vi "B Spline Fitting Demo.vi"() -> ()   [LabVIEW 2023]
doc: "This example generates data sets and then uses the B-Spline Fit VI (or its subVI) to create a best fit curve for the data. A best fit curve is generated each time you change the value of any of the controls."
uses:
  <vilib>/Native 3D Graph/xcontrol/3DPC_SurfacePlot.xctl
  <vilib>/Analysis/1siggen.llb/Ramp Pattern by Samples.vi
  <vilib>/Analysis/6fits.llb/1D B-Spline Fit.vi
  <vilib>/Analysis/6fits.llb/nD B-Spline Fit.vi
  <vilib>/Analysis/NI_AALBase.lvlib
  <vilib>/Analysis/NI_AALPro.lvlib
panel:
  in  "example selector":T1(tab)
  in  "parameter selection":u16(ring)=2 items=["equally spaced", "chord length", "centripetal"]
  in  "degree":i32=3
  in  "# of control points":i32=10
  out "1D B-Spline Fit on Arbitrary Curve":T2(graph)
  in  "# of control points":i32=30
  in  "degree":i32=7
  in  "parameter selection":u16(ring)=2 items=["equally spaced", "chord length", "centripetal"]
  in  "noise amplitude":dbl=0.01
  out "1D B-Spline Fit on Square Curve":T2(graph)
  out "B-Spline Fitted Curve":refnum<class "Base Datatype.lvclass">[](xcontrol)
  out "Original Curve":refnum<class "Base Datatype.lvclass">[](xcontrol)
  in  "noise amplitude":dbl=0.5
  in  "parameter selection":u16(ring)=2 items=["equally spaced", "chord length", "centripetal"]
  in  "degree":i32=3
  in  "# of control points":i32=15
  # "Overview: Demonstrates fitting curves with the B-Spline Fit VI.\nRequirements: LabVIEW Full Development System\nInstructions:\n1. Select a tab to specify which kind of fit to perform on which curve.\n2. Run the VI and observe the fit displayed on the graph.\n3. Select a different tab and run the VI again."
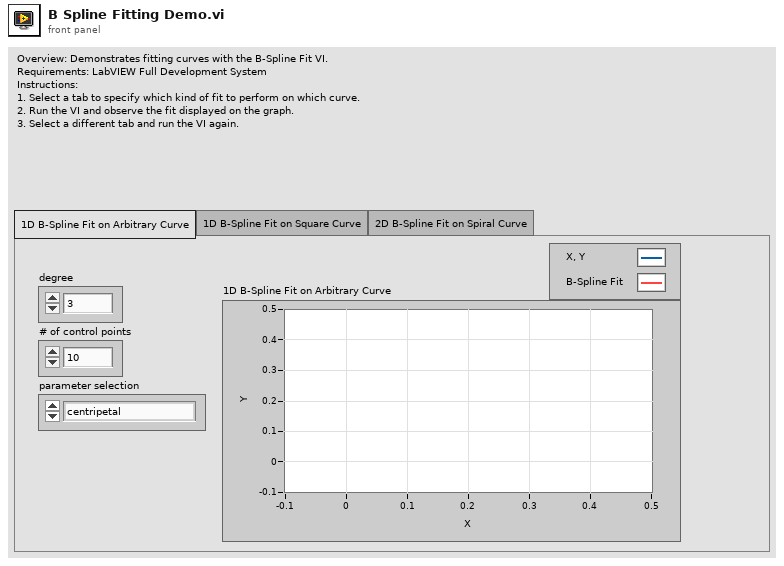
[diagram p1: front panel]
types:
  T1 = enum32{"1D B-Spline Fit on Arbitrary Curve", "1D B-Spline Fit on Square Curve", "2D B-Spline Fit on Spiral Curve"}
  T2 = cluster{"Best BSpline Fit X":dbl[], "Best BSpline Fit Y":dbl[]}[]
  T3 = cluster{"Best BSpline Fit X":dbl[], "Best BSpline Fit Y":dbl[]}
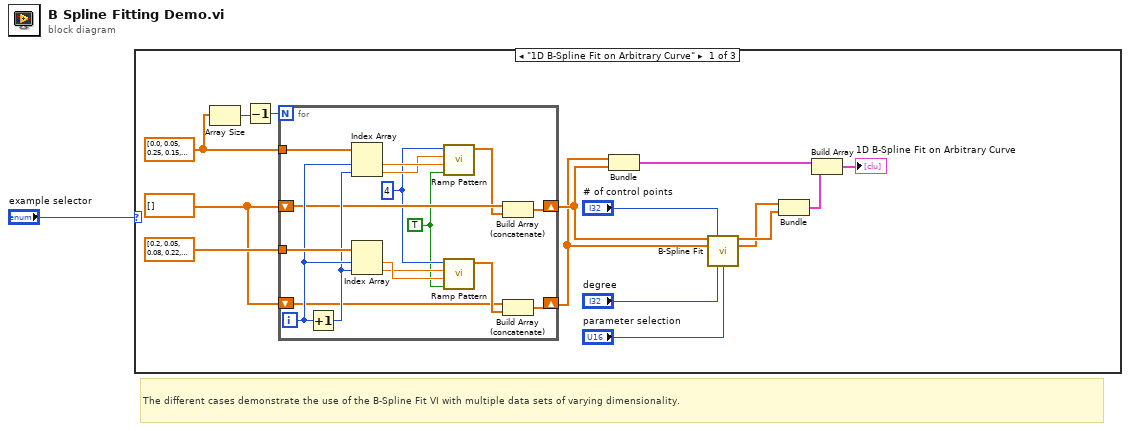
[diagram p0: block diagram]
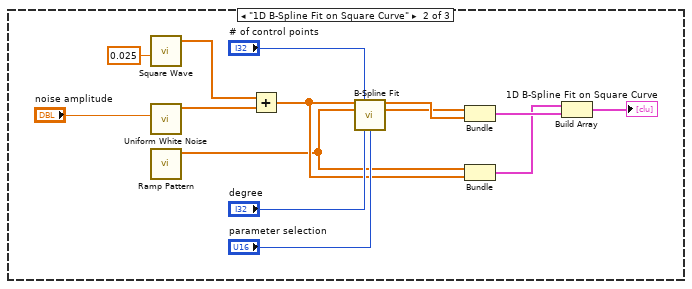
[diagram p2: hidden frame]
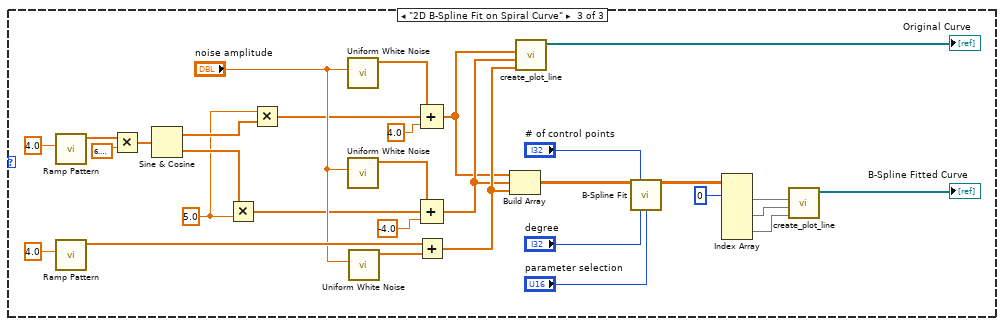
[diagram p3: hidden frame]
diagram:
  # "The different cases demonstrate the use of the B-Spline Fit VI with multiple data sets of varying dimensionality."
  n1 = case shown="\"1D B-Spline Fit on Arbitrary Curve\"" "example selector" {
    frame "1D B-Spline Fit on Arbitrary Curve" {
      w8 = dbl[] [0.0, 0.05, 0.25, 0.15, 0.0, 0.0, 0.35, 0.4, 0.3, 0.0] ("Y")
      w5 = dbl[] [] ("Y 2")
      n2 = Array Size(array=w8) -> (size(s)=w7:i32)
      n3 = Decrement(x=w7) -> (x-1=w6:i32)
      n4 = for {
        N: w6 -> [_]
        tunnel: w8 -> [w32]
        tunnel: dbl[] [0.2, 0.05, 0.08, 0.22, 0.3, 0.4, 0.35, 0.21, -0.05, 0.0] ("X") -> [w31]
        shift-right: [w25] -> w3
        shift-left: w5 -> [w26]
        shift-right: [w19] -> w2
        shift-left: w5 -> [w23]
        i -> [w30]
        w20 = 4 ("samples")
        w17 = TRUE ("exclude end?")
        n5 = Increment(x=w30) -> (x+1=w29:i32)
        n6 = Index Array(array=w32, index #1=w30, index #2=w29) -> (element #1=w28:dbl, element #2=w27:dbl)
        n7 = Index Array(array=w31, index #1=w30, index #2=w29) -> (element #1=w22:dbl, element #2=w21:dbl)
        n8 = call-poly <vilib>:"Ramp Pattern.vi"("exclude end?"=w17, "start"=w28, "end"=w27, "samples"=w20) -> ("Ramp Pattern"=w18:dbl[])  [unwired: 6 in, 1 out]
        n9 = call-poly <vilib>:"Ramp Pattern.vi"("exclude end?"=w17, "start"=w22, "end"=w21, "samples"=w20) -> ("Ramp Pattern"=w24:dbl[])  [unwired: 6 in, 1 out]
        n10 = Build Array (concatenate)(w26, w18) -> (w25:dbl[])
        n11 = Build Array (concatenate)(w23, w24) -> (w19:dbl[])
      }
      n12 = Bundle("Y 2"=w2, "Y 2"=w3) -> (w11:cluster{"Y 2":dbl[], "Y 2":dbl[]})  [unwired: 1 out]
      n13 = call-poly <vilib>:"B-Spline Fit.vi"("Y"=w3, "# of control points"="# of control points", "X"=w2, "degree"="degree", "parameter selection"="parameter selection") -> ("Best BSpline Fit Y"=w10:dbl[], "Best BSpline Fit X"=w4:dbl[])  [unwired: 7 in, 2 out]
      n14 = Bundle("Best BSpline Fit X"=w4, "Best BSpline Fit Y"=w10) -> (w12:T3)  [unwired: 1 out]
      n15 = Build Array(w11, w12) -> (→"1D B-Spline Fit on Arbitrary Curve":T2)
    }
    frame "1D B-Spline Fit on Square Curve" {
      n16 = call <vilib>:"Square Wave.vi"("frequency"=0.025) -> ("square wave"=w41:dbl[])  [unwired: 5 in, 2 out]
      n17 = call <vilib>:"Uniform White Noise.vi"("amplitude"="noise amplitude") -> ("uniform white noise"=w35:dbl[])  [unwired: 3 in, 7 out]
      n18 = call-poly <vilib>:"Ramp Pattern.vi"() -> ("Ramp Pattern"=w33:dbl[])  [unwired: 10 in, 1 out]
      n19 = Add(x=w41, y=w35) -> (x+y=w42:dbl[])
      n20 = call-poly <vilib>:"B-Spline Fit.vi"("Y"=w42, "# of control points"="# of control points", "X"=w33, "degree"="degree", "parameter selection"="parameter selection") -> ("Best BSpline Fit Y"=w38:dbl[], "Best BSpline Fit X"=w37:dbl[])  [unwired: 7 in, 2 out]
      n21 = Bundle("Best BSpline Fit X"=w37, "Best BSpline Fit Y"=w38) -> (w39:T3)  [unwired: 1 out]
      n22 = Bundle("Ramp Pattern"=w33, w42) -> (w36:cluster{"Ramp Pattern":dbl[], dbl[]})  [unwired: 1 out]
      n23 = Build Array(w36, w39) -> (→"1D B-Spline Fit on Square Curve":T2)
    }
    frame "2D B-Spline Fit on Spiral Curve" {
      w66 = 5.0 ("radius")
      n24 = call-poly <vilib>:"Ramp Pattern.vi"("end"=4.0) -> ("Ramp Pattern"=w71:dbl[])  [unwired: 9 in, 1 out]
      n25 = call-poly <vilib>:"Ramp Pattern.vi"("end"=4.0) -> ("Ramp Pattern"=w76:dbl[])  [unwired: 9 in, 1 out]
      n26 = Multiply(x=w71, y=6.283185307179586) -> (x*y=w69:dbl[])
      n27 = Sine & Cosine(0:w69) -> (1:w67:dbl[], 2:w68:dbl[])
      n28 = Multiply(x=w68, y=w66) -> (x*y=w54:dbl[])
      n29 = Multiply(x=w66, y=w67) -> (x*y=w55:dbl[])
      n30 = call <vilib>:"Uniform White Noise.vi"("amplitude"="noise amplitude") -> ("uniform white noise"=w72:dbl[])  [unwired: 3 in, 7 out]
      n31 = call <vilib>:"Uniform White Noise.vi"("amplitude"="noise amplitude") -> ("uniform white noise"=w73:dbl[])  [unwired: 3 in, 7 out]
      n32 = call <vilib>:"Uniform White Noise.vi"("amplitude"="noise amplitude") -> ("uniform white noise"=w77:dbl[])  [unwired: 3 in, 7 out]
      n33 = Add(x=w76, y=w77) -> (x+y=w63:dbl[])
      n34 = Compound Arithmetic op=ADD(w72, w55, 4.0 ("y-offset (b)")) -> (w61:dbl[])
      n35 = Compound Arithmetic op=ADD(w73, w54, -4.0 ("x-offset (a)")) -> (w62:dbl[])
      n36 = Build Array(w61, w62, w63) -> (w52:dbl[][])
      n37 = call <vilib>:"create_plot_line.vi"("z vector"=w63, "y vector"=w62, "x vector"=w61) -> ("plots out"=→"Original Curve":refnum<class "Base Datatype.lvclass">[])  [unwired: 2 in, 6 out]
      n38 = call-poly <vilib>:"B-Spline Fit.vi"("Data"=w52, "# of control points"="# of control points", "degree"="degree", "parameter selection"="parameter selection") -> ("Best BSpline Fit"=w51:dbl[][])  [unwired: 9 in, 2 out]
      n39 = Index Array(array=w51, index (row) #1=0 ("index (row)")) -> (element #1=w59:dbl[], element #2=w58:dbl[], element #3=w57:dbl[])  [unwired: 5 in]
      n40 = call <vilib>:"create_plot_line.vi"("z vector"=w57, "y vector"=w58, "x vector"=w59) -> ("plots out"=→"B-Spline Fitted Curve":refnum<class "Base Datatype.lvclass">[])  [unwired: 2 in, 6 out]
    }
  }
